vi "Export.vi"(8 "error in (no error)":errorcluster, 10 "Export Path":path, 11 "Project Path":path) -> (0 "error out":errorcluster, 3 "Ran?":bool)   [LabVIEW 2025, in "Project.lvclass"]
uses:
  Project.lvclass
  Elemental IO Properties.ctl
  Project.lvclass/Project.ctl
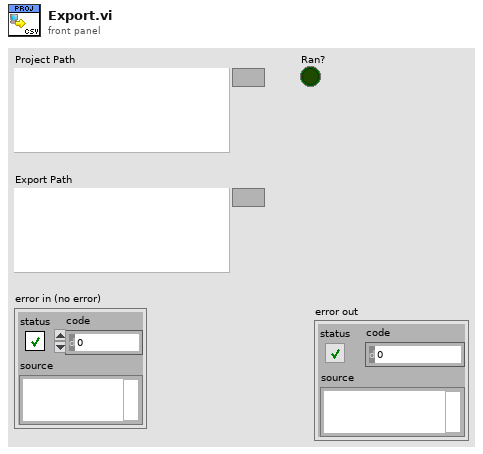
[diagram p1: front panel]
types:
  T1 = enum16{"open", "replace", "create", "open or create", "replace or create", "replace or create with confirmation"}
  T2 = typedef "Project.lvclass/Elemental IO Properties.ctl" = cluster{"FPGA Name":string, "Group":string, "IO Resource":string, "IO Name":string, "FPGA Resource":string}
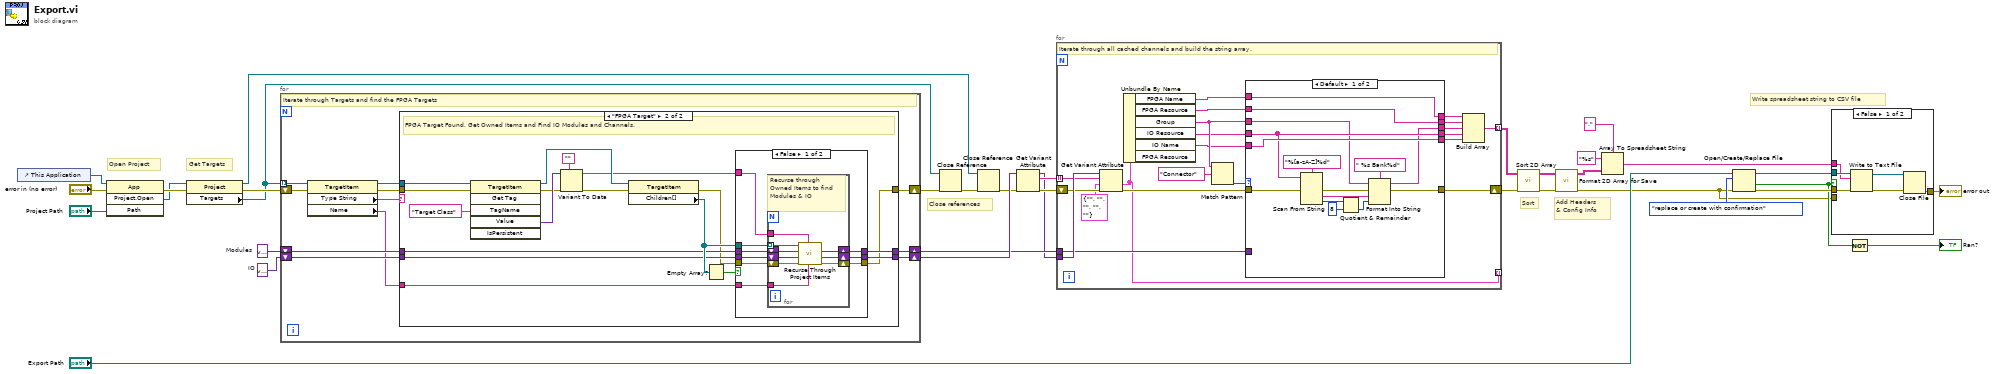
[diagram p0: block diagram]
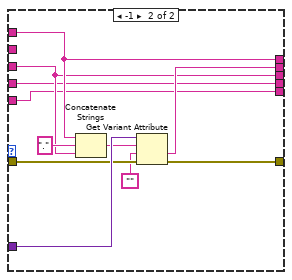
[diagram p5: hidden frame]
diagram:
  w25 = variant  # IO
  w26 = variant  # Modules
  # "Write spreadsheet string to CSV file"
  # "Add Headers \n& Config Info"
  # "Sort"
  # "Close references"
  # "Get Targets"
  # "Open Project"
  n1 = control-ref of="This Application"() -> (w34:refnum<vi>)
  n2 = invoke class="App" method="Project.Open"(reference=w34, error in="error in (no error)", "Path"="Project Path") -> (error out=w33:errorcluster, "Project:Open"=w32:refnum<vi>)  [unwired: 1 in, 2 out]
  n3 = property class="Project"(reference=w32, error in=w33) -> (reference out=w28:refnum<vi>, error out=w31:errorcluster, "Targets"=w29:refnum<vi>[])
  n4 = for {
    tunnel: w29 -> [w45] mode=indexing
    shift-right: [w42] -> w30
    shift-left: w31 -> [w44]
    shift-right: [w39] -> w22
    shift-left: w26 -> [w40]
    shift-right: [w37] -> w23
    shift-left: w25 -> [w38]
    # "Iterate through Targets and find the FPGA Targets"
    n5 = property class="TargetItem"(reference=w45, error in=w44) -> (reference out=w41:refnum<vi>, error out=w43:errorcluster, "Type String"=w36:string, "Name"=w35:string)
    n6 = case shown="\"FPGA Target\"" w36 {
      tunnel: w43 -> [w48 w56]
      tunnel: [w48 w58] -> w42
      tunnel: w41 -> [_ w55]
      tunnel: w40 -> [w47 w64]
      tunnel: w35 -> [_ w63]
      tunnel: [w47 w62] -> w39
      tunnel: w38 -> [w46 w61]
      tunnel: [w46 w60] -> w37
      frame "False", Default {
      }
      frame "FPGA Target" {
        # "FPGA Target Found, Get Owned Items and Find IO Modules and Channels."
        n7 = invoke class="TargetItem" method="Get Tag"(reference=w55, error in=w56, "TagName"="Target Class" ("Tag Name")) -> (reference out=w54:refnum<vi>, error out=w52:errorcluster, "Value"=w53:variant)  [unwired: 3 in, 3 out]
        n8 = Variant To Data(error in=w52, type="", Variant=w53) -> (data=w49:string, error out=w51:errorcluster)
        n9 = property class="TargetItem"(reference=w54, error in=w51) -> (error out=w59:errorcluster, "Children[]"=w66:refnum<vi>[])  [unwired: 1 out]
        n10 = Empty Array?(array=w66) -> (empty?=w65:bool)
        n11 = case shown="False" w65 {
          tunnel: w66 -> [w75 _]
          tunnel: w59 -> [w74 w85]
          tunnel: w64 -> [w73 w87]
          tunnel: w63 -> [w72 _]
          tunnel: [w71 w87] -> w62
          tunnel: w61 -> [w70 w86]
          tunnel: [w69 w86] -> w60
          tunnel: [w68 w85] -> w58
          tunnel: w49 -> [w67 _]
          frame False {
            n12 = for {
              tunnel: w75 -> [w84] mode=indexing
              shift-right: [w82] -> w68
              shift-left: w74 -> [w83]
              shift-right: [w81] -> w71
              shift-left: w73 -> [w78]
              tunnel: w72 -> [w77]
              shift-right: [w80] -> w69
              shift-left: w70 -> [w79]
              tunnel: w67 -> [w76]
              # "Recurse through Owned Items to find Modules & IO"
              n13 = call "Recurse Through Project Items.vi"("FPGA"=w77, "FPGA Resource"=w76, "error in (no error)"=w83, "IO in"=w79, "Modules in"=w78, "ProjectItem in"=w84) -> ("error out"=w82:errorcluster, "IO out"=w80:variant, "Modules out"=w81:variant)  [unwired: 3 in]
            }
          }
          frame True {
          }
        }
      }
    }
  }
  n14 = Close Reference(reference=w29, error in (no error)=w30) -> (error out=w27:errorcluster)
  n15 = Close Reference(reference=w28, error in (no error)=w27) -> (error out=w20:errorcluster)
  n16 = Get Variant Attribute(Variant=w23, error in=w20) -> (duplicate Variant=w19:variant, names=w24:string[], error out=w21:errorcluster)  [unwired: 2 in, 1 out]
  n17 = for {
    tunnel: w24 -> [w101] mode=indexing
    tunnel: w19 -> [w108]
    tunnel: w22 -> [w107]
    tunnel: [w103] -> w4 mode=indexing
    shift-right: [w102] -> w9
    shift-left: w21 -> [w105]
    tunnel: [w88] -> _ mode=indexing
    # "Iterate through all cached channels and build the string array."
    n18 = Get Variant Attribute(Variant=w108, name=w101, default value (empty Variant)=T2 {"FPGA Name"="", "Group"="", "IO Resource"="", "IO Name"="", "FPGA Resource"=""}, error in=w105) -> (value=w88:T2, error out=w106:errorcluster)  [unwired: 2 out]
    n19 = Unbundle By Name(w88) -> ("FPGA Name"=w104:string, "FPGA Resource"=w89:string, "Group"=w98:string, "IO Resource"=w93:string, "IO Name"=w90:string)  [unwired: 1 out]
    n20 = Match Pattern(string=w98, regular expression="Connector") -> (offset past match=w96:i32)  [unwired: 1 in, 3 out]
    n21 = case shown="Default" w96 {
      tunnel: w107 -> [_ w134]
      tunnel: w106 -> [w120 w132]
      tunnel: w104 -> [w122 w127]
      tunnel: [w115 w131] -> w102
      tunnel: [w110 w128] -> w99
      tunnel: w98 -> [w114 w126]
      tunnel: [w122 w127] -> w95
      tunnel: [w109 w126] -> w94
      tunnel: w93 -> [w119 w125]
      tunnel: [w119 w125] -> w92
      tunnel: [w123 w124] -> w91
      tunnel: w90 -> [w123 w124]
      tunnel: w89 -> [w110 _]
      frame Default {
        n22 = Scan From String(format string="%[a-zA-Z]%d", input string=w119, error in=w120) -> (error out=w116:errorcluster, output 1=w112:string, output 2=w118:i32)  [unwired: 3 in, 2 out]
        n23 = Quotient & Remainder(x=w118, y=8) -> (floor(x/y)=w111:i32)  [unwired: 1 out]
        n24 = Format Into String(format string=" %s Bank%d", initial string=w114, error in=w116, w112, w111) -> (resulting string=w109:string, error out=w115:errorcluster)
      }
      frame -1 {
        n25 = Concatenate Strings(w127, "." ("string"), w126) -> (w130:string)
        n26 = Get Variant Attribute(Variant=w134, name=w130, default value (empty Variant)="", error in=w132) -> (value=w128:string, error out=w131:errorcluster)  [unwired: 2 out]
      }
    }
    n27 = Build Array(w95, w99, w94, w92, w91) -> (w103:string[])
  }
  n28 = call "Sort 2D Array.vi"("error in (no error)"=w9, "Array in"=w4) -> ("error out"=w5:errorcluster, "Array out"=w7:string[][])  [unwired: 8 in]
  n29 = call "Format 2D Array for Save.vi"("error in (no error)"=w5, "Signals"=w7) -> ("error out"=w2:errorcluster, "Formated Table"=w6:string[][])  [unwired: 8 in]
  n30 = Array To Spreadsheet String(delimiter (Tab)=",", array=w6, 3:"%s" ("format string")) -> (spreadsheet string=w12:string)
  n31 = Open/Create/Replace File(file path (use dialog)="Export Path", error in=w2, operation (0:open)=T1."replace or create with confirmation") -> (refnum out=w14:refnum<file>, cancelled=w3:bool, error out=w15:errorcluster)  [unwired: 3 in]
  n32 = case shown="False" w3 {
    tunnel: w15 -> [w140 _]
    tunnel: w14 -> [w139 _]
    tunnel: w12 -> [w136 _]
    tunnel: [w135 w141] -> w11
    tunnel: w2 -> [_ w141]
    frame False {
      n33 = Write to Text File(file (use dialog)=w139, text=w136, error in=w140) -> (refnum out=w137:refnum<file>, error out=w138:errorcluster)  [unwired: 1 in, 1 out]
      n34 = Close File(refnum=w137, error in=w138) -> (error out=w135:errorcluster)  [unwired: 1 out]
    }
    frame True {
    }
  }
  "error out" <- w11
  n35 = Not(x=w3) -> (.not. x?=→"Ran?":bool)
